vi "Other Vision VI.vi"(7 "error in":errorcluster) -> (20 "Straight Edge (Find Straight Edge 1)":T2 {"Point2 (Real-World)"."Y" format="%.2f"; "Point2 (Real-World)"."X" format="%.2f"; "Point1 (Real-World)"."Y" format="%.2f"; "Point1 (Real-World)"."X" format="%.2f"; "Point2 (Pixels)"."Y" format="%.2f"; "Point2 (Pixels)"."X" format="%.2f"; "Point1 (Pixels)"."Y" format="%.2f"; "Point1 (Pixels)"."X" format="%.2f"}, 21 "Straight Edge (Find Straight Edge 2)":T2 {"Point2 (Real-World)"."Y" format="%.2f"; "Point2 (Real-World)"."X" format="%.2f"; "Point1 (Real-World)"."Y" format="%.2f"; "Point1 (Real-World)"."X" format="%.2f"; "Point2 (Pixels)"."Y" format="%.2f"; "Point2 (Pixels)"."X" format="%.2f"; "Point1 (Pixels)"."Y" format="%.2f"; "Point1 (Pixels)"."X" format="%.2f"}, 22 "Straight Edge (Find Straight Edge 3)":T2 {"Point2 (Real-World)"."Y" format="%.2f"; "Point2 (Real-World)"."X" format="%.2f"; "Point1 (Real-World)"."Y" format="%.2f"; "Point1 (Real-World)"."X" format="%.2f"; "Point2 (Pixels)"."Y" format="%.2f"; "Point2 (Pixels)"."X" format="%.2f"; "Point1 (Pixels)"."Y" format="%.2f"; "Point1 (Pixels)"."X" format="%.2f"}, 27 "error out":errorcluster)   [LabVIEW 2014]
uses:
  <vilib>/vision/Measure.llb/Edge Options.ctl
  <vilib>/vision/Measure.llb/Edge Polarity.ctl
  <vilib>/vision/Measure.llb/Straight Edge Options.ctl
  <vilib>/vision/Measure.llb/Straight Edge Process.ctl
  <vilib>/vision/NI_Vision_Development_Module.lvlib
panel:
  out "Image Out":T1(plugin-control)
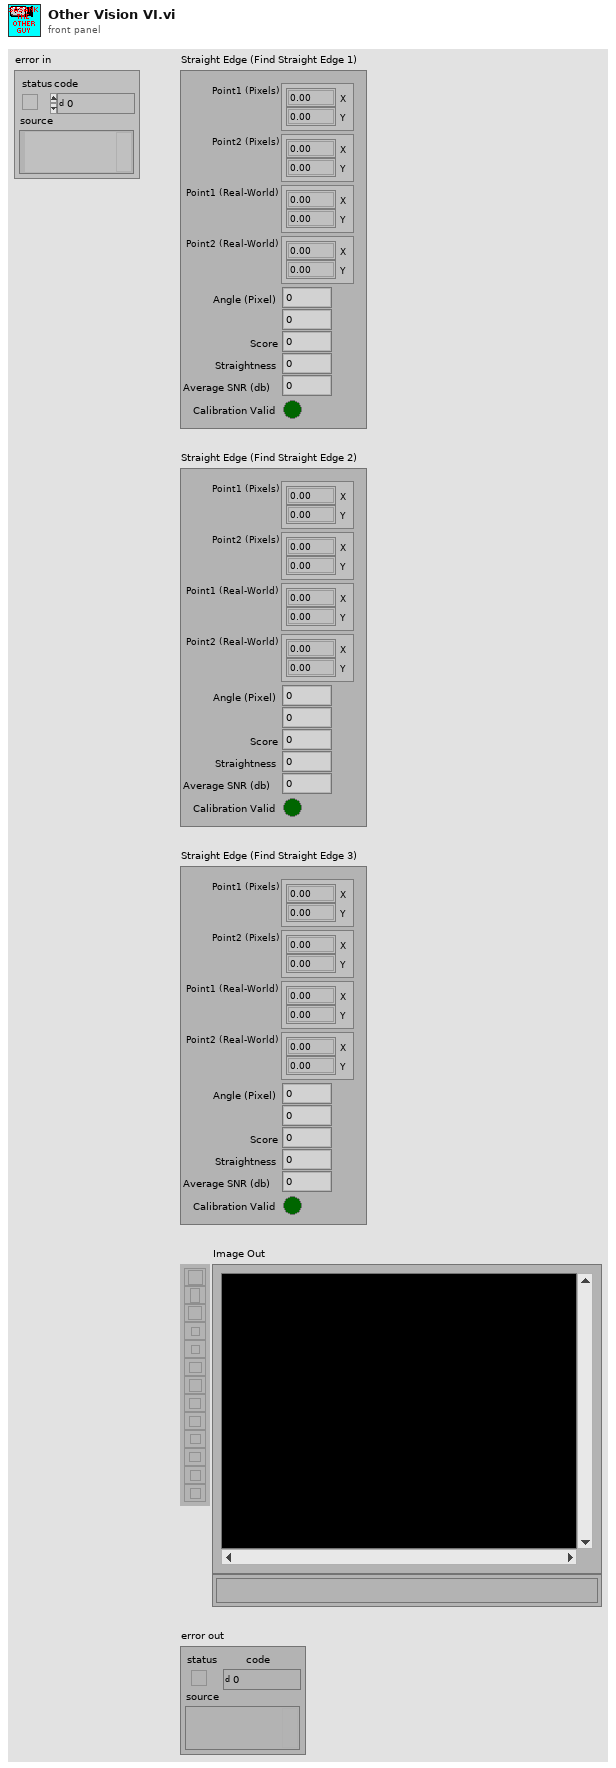
[diagram p1: front panel]
types:
  T1 = typedef "IMAQ Image.ctl" = refnum<image>
  T2 = cluster{"Point1 (Pixels)":cluster{"X":sgl, "Y":sgl}, "Point2 (Pixels)":cluster{"X":sgl, "Y":sgl}, "Point1 (Real-World)":cluster{"X":sgl, "Y":sgl}, "Point2 (Real-World)":cluster{"X":sgl, "Y":sgl}, "Angle (Pixel)":dbl, "Angle (Real-World)":dbl, "Score":dbl, "Straightness":dbl, "Average SNR (db)":dbl, "Calibration Valid":bool}
  T3 = typedef "Edge Options.ctl" = cluster{"Edge Polarity":T4, "Kernel Size":u32, "Width":u32, "Minimum Edge Strength":sgl, "Interpolation Type":enum32{"Zero Order", "Bilinear", "Quadratic", "Cubic", "Bilinear Fixed"}, "Data Processing Method":enum32{"Average", "Median"}}
  T4 = typedef "Edge Polarity.ctl" = u32
  T5 = cluster{"Search Direction":u32, "Edge Options":T3, "Show Search Area":bool, "Show Search Lines":bool, "Show Edges Found":bool, "Show Result":bool, "Search Area Color":u32, "Search Lines Color":u32, "Edge Locations Color":u32, "Result Color":u32, "Overlay Group Name":string}
  T6 = typedef "Straight Edge Options.ctl" = cluster{"Number of Lines":i32, "Type":T7, "Min. Score":dbl, "Max. Score":dbl, "Orientation":dbl, "Angle Range":dbl, "Angle Tolerance":dbl, "Step Size":u32, "Min. SNR (db)":dbl, "Min. Points (%)":dbl, "Hough Iterations":i32}
  T7 = typedef "Straight Edge Process.ctl" = enum32{"First Edge Rake", "Best Edge Rake", "Hough Edge Rake", "First Edge Projection", "Best Edge Projection"}
  T8 = cluster{"Global Rectangle":i32[], "Contours":cluster{"ID":enum32{"External", "Internal"}, "Type":u32, "Coordinates":i32[]}[]}
  T9 = cluster{"Measurement Parameter":i32, "Range Lower Value":dbl, "Range Upper Value":dbl, "Range":bool, "Measurement Type":bool}[]
  T10 = enum32{"Linear", "Log", "Exp", "Square", "Square root", "Power X", "Power 1/X"}
  T11 = cluster{"Brightness":sgl, "Contrast":sgl, "Gamma":sgl}
  T12 = typedef "Image Type" = u32
  T13 = cluster{"histogram":u32[], "Minimal Value":sgl, "Maximal Value":sgl, "Starting Value":sgl, "Interval Width":sgl, "Mean Value":sgl, "Standard  Variation":sgl, "Area (pixels)":i32}
  T14 = cluster{"Point1 (Pixels)":cluster{"X":sgl, "Y":sgl}, "Point2 (Pixels)":cluster{"X":sgl, "Y":sgl}, "Point1 (Real-World)":cluster{"X":sgl, "Y":sgl}, "Point2 (Real-World)":cluster{"X":sgl, "Y":sgl}, "Angle (Pixel)":dbl, "Angle (Real-World)":dbl, "Score":dbl, "Straightness":dbl, "Average SNR (db)":dbl, "Calibration Valid":bool}[]
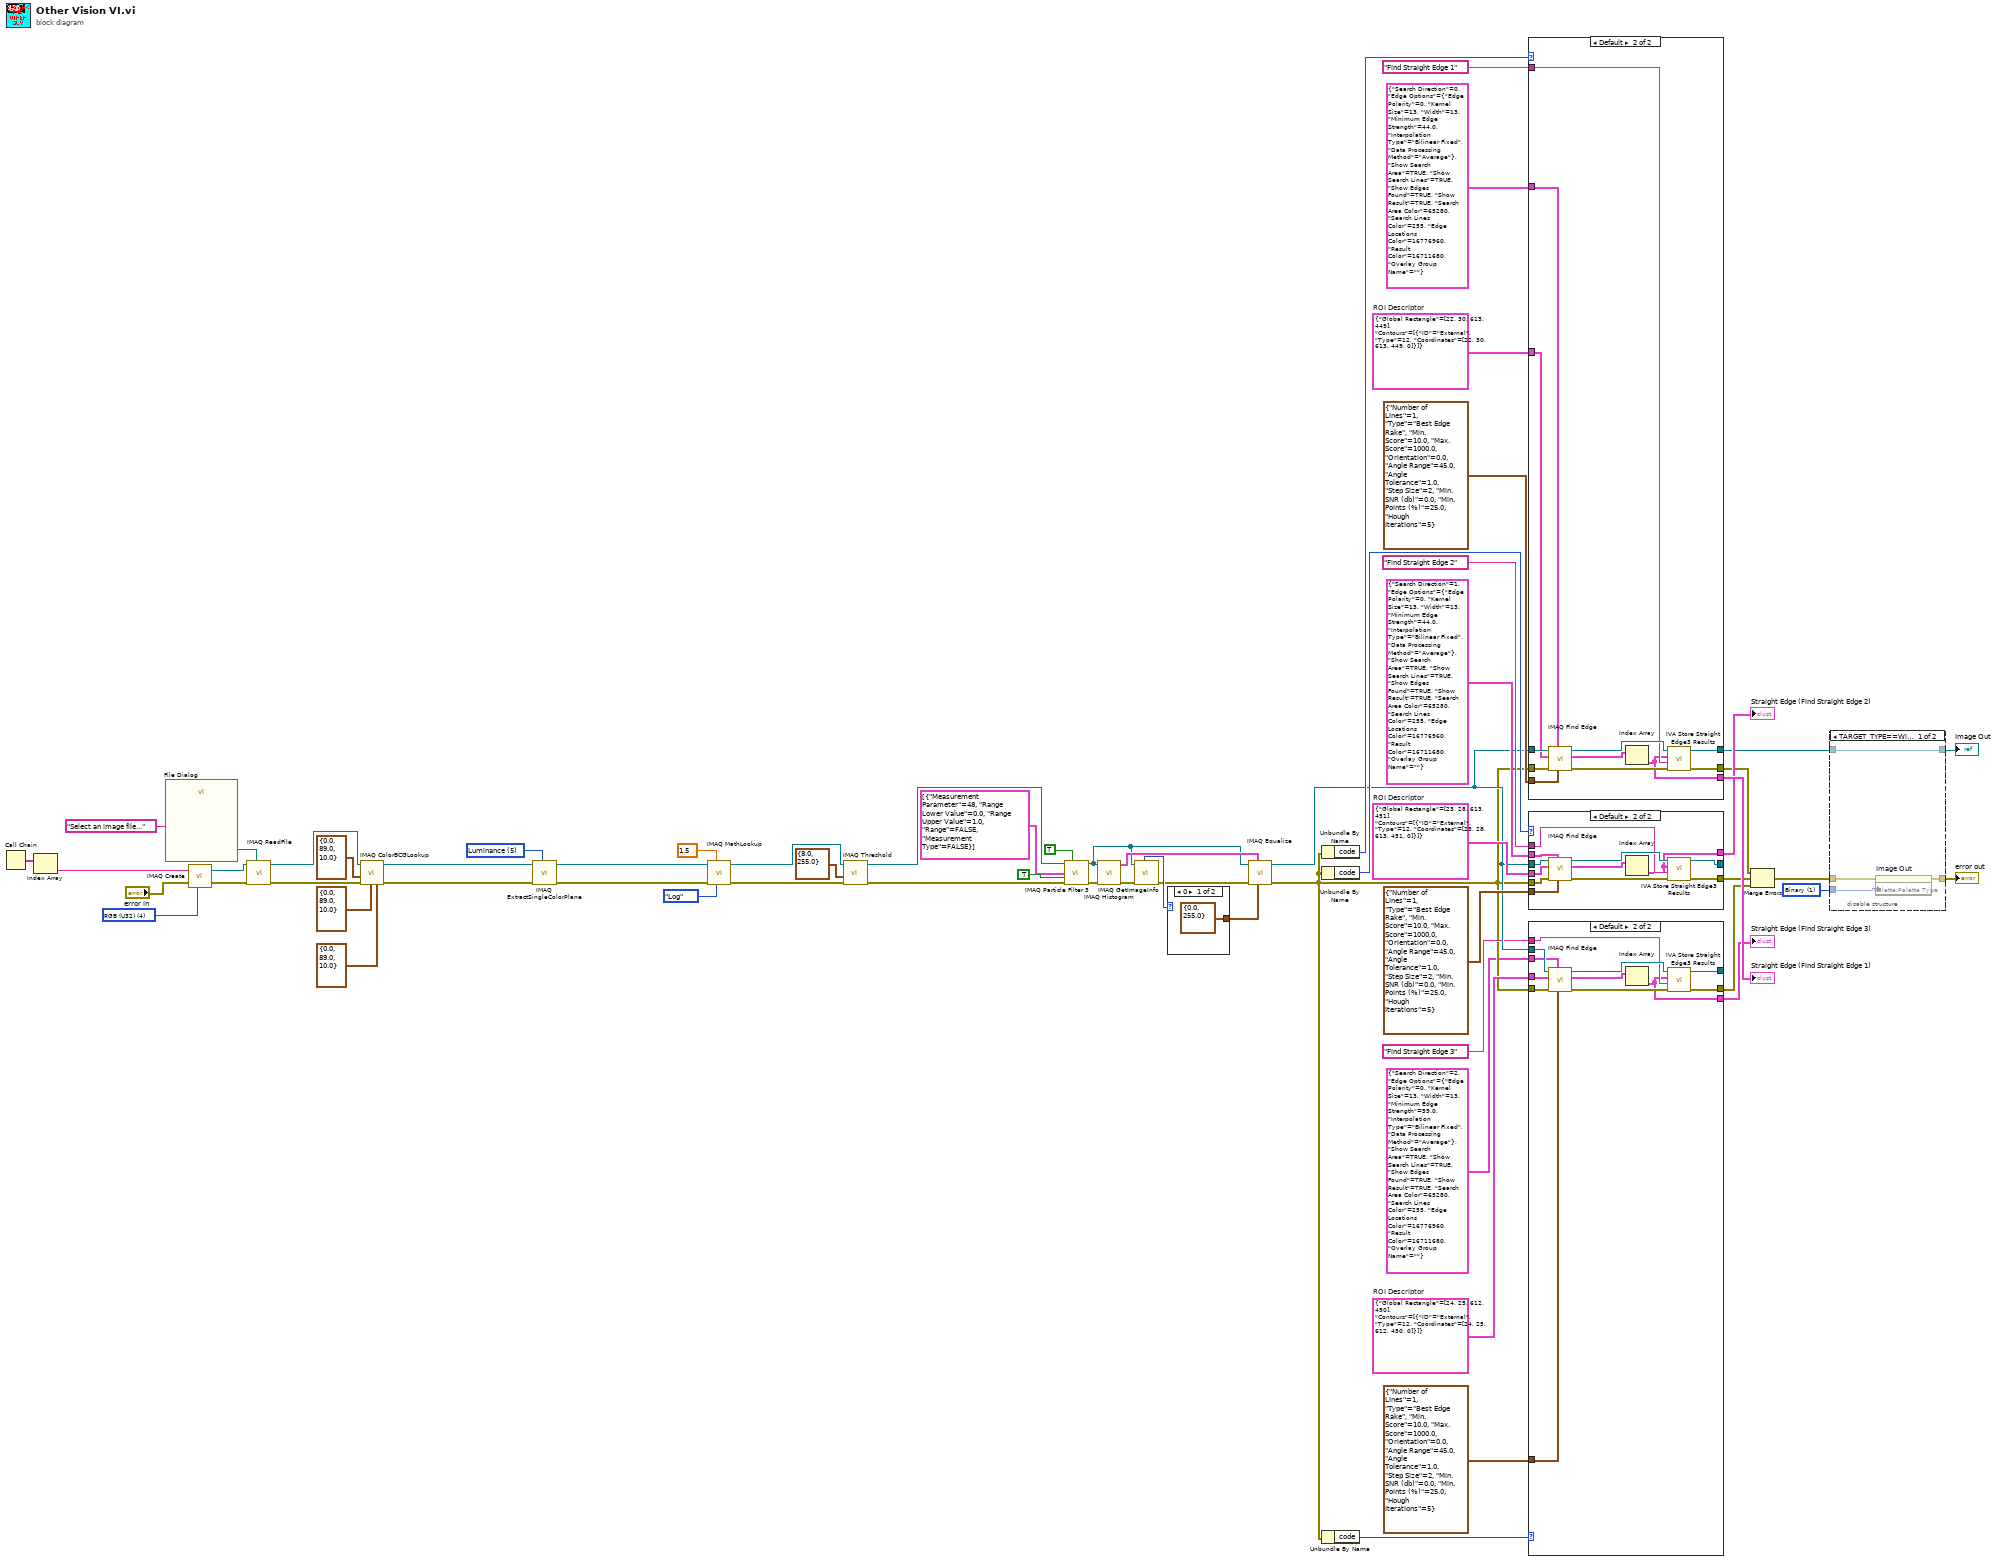
[diagram p0: block diagram]
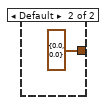
[diagram p6: hidden frame]
diagram:
  w1 = u32 1 items=["Grayscale", "Binary", "Gradient", "Rainbow", "Temperature", "User Defined"] ("Palette")
  w15 = T8 {"Global Rectangle"=[24, 25, 612, 450], "Contours"=[{"ID"=enum."External", "Type"=12, "Coordinates"=[24, 25, 612, 450, 0]}]}  # ROI Descriptor
  w22 = T8 {"Global Rectangle"=[23, 28, 613, 451], "Contours"=[{"ID"=enum."External", "Type"=12, "Coordinates"=[23, 28, 613, 451, 0]}]}  # ROI Descriptor
  w28 = T8 {"Global Rectangle"=[22, 30, 613, 449], "Contours"=[{"ID"=enum."External", "Type"=12, "Coordinates"=[22, 30, 613, 449, 0]}]}  # ROI Descriptor
  w50 = 5 items=["Red", "Green", "Blue", "Hue", "Saturation", "Luminance", "Value", "Intensity"] ("Color Plane")
  w56 = T12 4 items=["Grayscale (U8)", "Grayscale (I16)", "Grayscale (SGL)", "Complex (CSG)", "RGB (U32)", "HSL (U32)", "RGB (U64)", "Grayscale (U16)"] ("Image Type")
  n1 = Call Chain() -> (call chain=w60:string[])
  n2 = Index Array(array=w60) -> (element=w59:string)  [unwired: 1 in]
  n3 = call "File Dialog"("prompt"="Select an image file...") -> ("selected path"=w57:path)  [unwired: 6 in, 8 out]
  n4 = call "IMAQ Create"("Image Name"=w59, "Image Type"=w56, "error in (no error)"="error in") -> ("New Image"=w63:T1, "error out"=w62:errorcluster)  [unwired: 1 in, 1 out]
  n5 = call "IMAQ ReadFile"("File Path"=w57, "error in (no error)"=w62, "Image"=w63) -> ("error out"=w54:errorcluster, "Image Out"=w55:T1)  [unwired: 2 in, 5 out]
  n6 = call "IMAQ ColorBCGLookup"("Blue BCG Values"=T11 {"Brightness"=0.0, "Contrast"=89.0, "Gamma"=10.0}, "Green BCG Values"=T11 {"Brightness"=0.0, "Contrast"=89.0, "Gamma"=10.0}, "error in (no error)"=w54, "Red BCG Values"=T11 {"Brightness"=0.0, "Contrast"=89.0, "Gamma"=10.0}, "Image Src"=w55) -> ("error out"=w48:errorcluster, "Image Dst Out"=w49:T1)  [unwired: 2 in, 3 out]
  n7 = call "IMAQ ExtractSingleColorPlane"("Color Plane"=w50, "error in (no error)"=w48, "Image Src"=w49) -> ("error out"=w44:errorcluster, "Image Dst Out"=w45:T1)  [unwired: 1 in, 6 out]
  n8 = call "IMAQ MathLookup"("Operator"=T10."Log", "X Value"=sgl 1.5, "error in (no error)"=w44, "Image Src"=w45) -> ("error out"=w41:errorcluster, "Image Dst Out"=w42:T1)  [unwired: 3 in, 3 out]
  n9 = call "IMAQ Threshold"("error in (no error)"=w41, "Range"=cluster{"Lower value":sgl, "Upper value":sgl} {"Lower value"=8.0, "Upper value"=255.0}, "Image Src"=w42) -> ("error out"=w37:errorcluster, "Image Dst Out"=w38:T1)  [unwired: 3 in, 4 out]
  n10 = call "IMAQ Particle Filter 3"("Image Src"=w38, "Connectivity 4/8 (8)"=TRUE, "Selection Values"=T9 [{"Measurement Parameter"=48, "Range Lower Value"=0.0, "Range Upper Value"=1.0, "Range"=FALSE, "Measurement Type"=FALSE}], "Keep/Remove Particles (F)"=TRUE ("Keep/Remove Particles"), "error in (no error)"=w37) -> ("Image Dst Out"=w32:T1, "error out"=w34:errorcluster)  [unwired: 4 in, 5 out]
  n11 = call "IMAQ Histogram"("error in (no error)"=w34, "Image"=w32) -> ("error out"=w31:errorcluster, "Histogram Report"=w35:T13)  [unwired: 3 in, 5 out]
  n12 = call "IMAQ GetImageInfo"("error in (no error)"=w31, "Image"=w32) -> ("error out"=w30:errorcluster, "Image Type"=w33:T12)  [unwired: 8 out]
  n13 = case shown="0" w33 {
    tunnel: [cluster{"Minimum":sgl, "Maximum":sgl} {"Minimum"=0.0, "Maximum"=255.0} ("Range") cluster{"Minimum":sgl, "Maximum":sgl} {"Minimum"=0.0, "Maximum"=0.0} ("Range")] -> w29
    frame 0 {
    }
    frame Default {
    }
  }
  n14 = call "IMAQ Equalize"("Range"=w29, "Histogram Report"=w35, "error in (no error)"=w30, "Image Src"=w32) -> ("error out"=w13:errorcluster, "Image Dst Out"=w16:T1)  [unwired: 2 in, 4 out]
  n15 = Unbundle By Name(w13) -> ("code"=w26:i32)
  n16 = Unbundle By Name(w13) -> ("code"=w20:i32)
  n17 = Unbundle By Name(w13) -> ("code"=w12:i32)
  n18 = case shown="Default" w26 {
    tunnel: w16 -> [w66 w78]
    tunnel: w13 -> [_ w77]
    tunnel: w28 -> [_ w71]
    tunnel: [w66 w75] -> w3
    tunnel: [_ w73] -> w8
    tunnel: "Find Straight Edge 1" ("Step Name") -> [_ w72]
    tunnel: T6 {"Number of Lines"=1, "Type"=enum."Best Edge Rake", "Min. Score"=10.0, "Max. Score"=1000.0, "Orientation"=0.0, "Angle Range"=45.0, "Angle Tolerance"=1.0, "Step Size"=2, "Min. SNR (db)"=0.0, "Min. Points (%)"=25.0, "Hough Iterations"=5} ("Fit Options") -> [_ w70]
    tunnel: T5 {"Search Direction"=0, "Edge Options"={"Edge Polarity"=0, "Kernel Size"=13, "Width"=13, "Minimum Edge Strength"=44.0, "Interpolation Type"=enum."Bilinear Fixed", "Data Processing Method"=enum."Average"}, "Show Search Area"=TRUE, "Show Search Lines"=TRUE, "Show Edges Found"=TRUE, "Show Result"=TRUE, "Search Area Color"=65280, "Search Lines Color"=255, "Edge Locations Color"=16776960, "Result Color"=16711680, "Overlay Group Name"=""} ("Options") -> [_ w69]
    tunnel: [_ w67] -> w23
    frame -1074396199, -1074396198 {
      # "Discard Coordinate System Error"
    }
    frame Default {
      n19 = call "IMAQ Find Edge"("Line Fit Options"=w70, "Options"=w69, "error in (no error)"=w77, "ROI Descriptor"=w71, "Image"=w78) -> ("error out"=w74:errorcluster, "Straight Edges"=w68:T14, "Image Out"=w76:T1)  [unwired: 1 in, 3 out]
      n20 = Index Array(array=w68) -> (element=w67:T2)  [unwired: 1 in]
      n21 = call <vilib>:"IVA Store Straight Edge3 Results.vi"("error in (no error)"=w74, "Step Name"=w72, "Straight Edge"=w67, "Image in"=w76) -> ("error out"=w73:errorcluster, "Image dup"=w75:T1)  [unwired: 1 in, 5 out]
    }
  }
  "Straight Edge (Find Straight Edge 1)" <- w23
  n22 = case shown="Default" w20 {
    tunnel: w16 -> [w79 w91]
    tunnel: w13 -> [_ w90]
    tunnel: w22 -> [_ w84]
    tunnel: [w79 w88] -> _
    tunnel: [_ w86] -> w7
    tunnel: "Find Straight Edge 2" ("Step Name") -> [_ w85]
    tunnel: T6 {"Number of Lines"=1, "Type"=enum."Best Edge Rake", "Min. Score"=10.0, "Max. Score"=1000.0, "Orientation"=0.0, "Angle Range"=45.0, "Angle Tolerance"=1.0, "Step Size"=2, "Min. SNR (db)"=0.0, "Min. Points (%)"=25.0, "Hough Iterations"=5} ("Fit Options") -> [_ w83]
    tunnel: T5 {"Search Direction"=1, "Edge Options"={"Edge Polarity"=0, "Kernel Size"=13, "Width"=13, "Minimum Edge Strength"=44.0, "Interpolation Type"=enum."Bilinear Fixed", "Data Processing Method"=enum."Average"}, "Show Search Area"=TRUE, "Show Search Lines"=TRUE, "Show Edges Found"=TRUE, "Show Result"=TRUE, "Search Area Color"=65280, "Search Lines Color"=255, "Edge Locations Color"=16776960, "Result Color"=16711680, "Overlay Group Name"=""} ("Options") -> [_ w82]
    tunnel: [_ w80] -> w17
    frame -1074396199, -1074396198 {
      # "Discard Coordinate System Error"
    }
    frame Default {
      n23 = call "IMAQ Find Edge"("Line Fit Options"=w83, "Options"=w82, "error in (no error)"=w90, "ROI Descriptor"=w84, "Image"=w91) -> ("error out"=w87:errorcluster, "Straight Edges"=w81:T14, "Image Out"=w89:T1)  [unwired: 1 in, 3 out]
      n24 = Index Array(array=w81) -> (element=w80:T2)  [unwired: 1 in]
      n25 = call <vilib>:"IVA Store Straight Edge3 Results.vi"("error in (no error)"=w87, "Step Name"=w85, "Straight Edge"=w80, "Image in"=w89) -> ("error out"=w86:errorcluster, "Image dup"=w88:T1)  [unwired: 1 in, 5 out]
    }
  }
  "Straight Edge (Find Straight Edge 2)" <- w17
  n26 = case shown="Default" w12 {
    tunnel: w16 -> [w92 w104]
    tunnel: w13 -> [_ w103]
    tunnel: w15 -> [_ w97]
    tunnel: [w92 w101] -> _
    tunnel: [_ w99] -> w6
    tunnel: "Find Straight Edge 3" ("Step Name") -> [_ w98]
    tunnel: T6 {"Number of Lines"=1, "Type"=enum."Best Edge Rake", "Min. Score"=10.0, "Max. Score"=1000.0, "Orientation"=0.0, "Angle Range"=45.0, "Angle Tolerance"=1.0, "Step Size"=2, "Min. SNR (db)"=0.0, "Min. Points (%)"=25.0, "Hough Iterations"=5} ("Fit Options") -> [_ w96]
    tunnel: T5 {"Search Direction"=2, "Edge Options"={"Edge Polarity"=0, "Kernel Size"=13, "Width"=13, "Minimum Edge Strength"=59.0, "Interpolation Type"=enum."Bilinear Fixed", "Data Processing Method"=enum."Average"}, "Show Search Area"=TRUE, "Show Search Lines"=TRUE, "Show Edges Found"=TRUE, "Show Result"=TRUE, "Search Area Color"=65280, "Search Lines Color"=255, "Edge Locations Color"=16776960, "Result Color"=16711680, "Overlay Group Name"=""} ("Options") -> [_ w95]
    tunnel: [_ w93] -> w9
    frame -1074396199, -1074396198 {
      # "Discard Coordinate System Error"
    }
    frame Default {
      n27 = call "IMAQ Find Edge"("Line Fit Options"=w96, "Options"=w95, "error in (no error)"=w103, "ROI Descriptor"=w97, "Image"=w104) -> ("error out"=w100:errorcluster, "Straight Edges"=w94:T14, "Image Out"=w102:T1)  [unwired: 1 in, 3 out]
      n28 = Index Array(array=w94) -> (element=w93:T2)  [unwired: 1 in]
      n29 = call <vilib>:"IVA Store Straight Edge3 Results.vi"("error in (no error)"=w100, "Step Name"=w98, "Straight Edge"=w93, "Image in"=w102) -> ("error out"=w99:errorcluster, "Image dup"=w101:T1)  [unwired: 1 in, 5 out]
    }
  }
  "Straight Edge (Find Straight Edge 3)" <- w9
  n30 = Merge Errors(w8, w7, w6) -> (w5:errorcluster)
  n31 = disable-structure "Conditional Disable Structure" shown="TARGET_TYPE==Windows" {
    disable-tunnel: w5 -> [w108 w109]
    disable-tunnel: [w107 w109] -> w4
    disable-tunnel: w3 -> [w106 w110]
    disable-tunnel: [w106 w110] -> w2
    disable-tunnel: w1 -> [w105 _]
    frame condition #0 {
      n32 = property on="Image Out" class="ImageControl"(error in=w108, "Palette:Palette Type"=w105) -> (error out=w107:errorcluster)  [unwired: 1 in, 1 out]
    }
    frame condition #1 (active) {
    }
  }
  "error out" <- w4
  "Image Out" <- w2
